vi "0506_Identificador_de_cor.vi"() -> (27 "error out":errorcluster)   [LabVIEW 2017]
uses:
  <vilib>/userdefined/High Color/IMAQdx.ctl
  <vilib>/vision/driver/IMAQdx.llb/IMAQdx Acquisition Mode.ctl
  <vilib>/vision/Classification.llb/IMAQ Classifier Read Options.ctl
  <vilib>/vision/driver/IMAQdx.llb/IMAQdx Buffer Number Mode.ctl
  <vilib>/vision/driver/NI_Vision_Acquisition_Software.lvlib
  <vilib>/vision/NI_Vision_Development_Module.lvlib
panel:
  out "Class":string
  out "dt":dbl
  out "Image Out 2":T1(plugin-control)
  in  "Câmera":T2="cam1"
  in  "Stop Button":bool
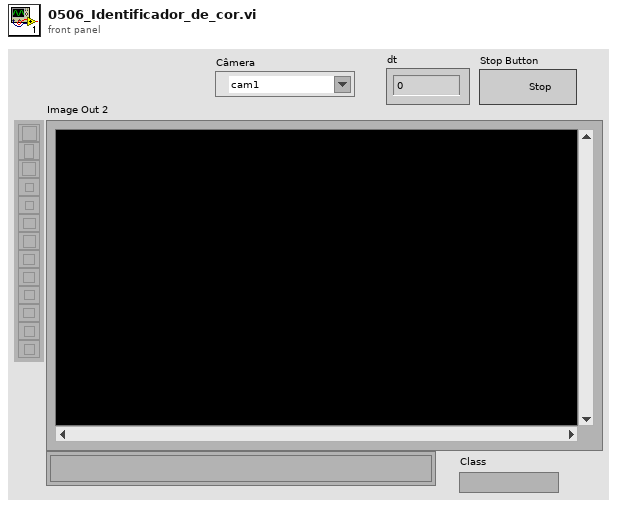
[diagram p1: front panel]
types:
  T1 = typedef "IMAQ Image.ctl" = refnum<image>
  T2 = typedef "IMAQdx.ctl" = refnum<k21>
  T3 = typedef "IMAQ Classifier Read Options.ctl" = i32
  T4 = typedef "Image Type" = u32
  T5 = typedef "NI_Vision_Acquisition_Software.lvlib/IMAQdx Acquisition Mode.ctl" = enum32{"One Shot", "Continuous"}
  T6 = typedef "IMAQ Classifier Session.ctl" = refnum<k1>
  T7 = typedef "NI_Vision_Acquisition_Software.lvlib/IMAQdx Buffer Number Mode.ctl" = enum32{"Next", "Last", "Buffer Number", "Every", "Last New"}
  T8 = cluster{"Global Rectangle":i32[], "Contours":cluster{"Contour Type":u32, "ROI Type":u32, "Points":i32[]}[]}
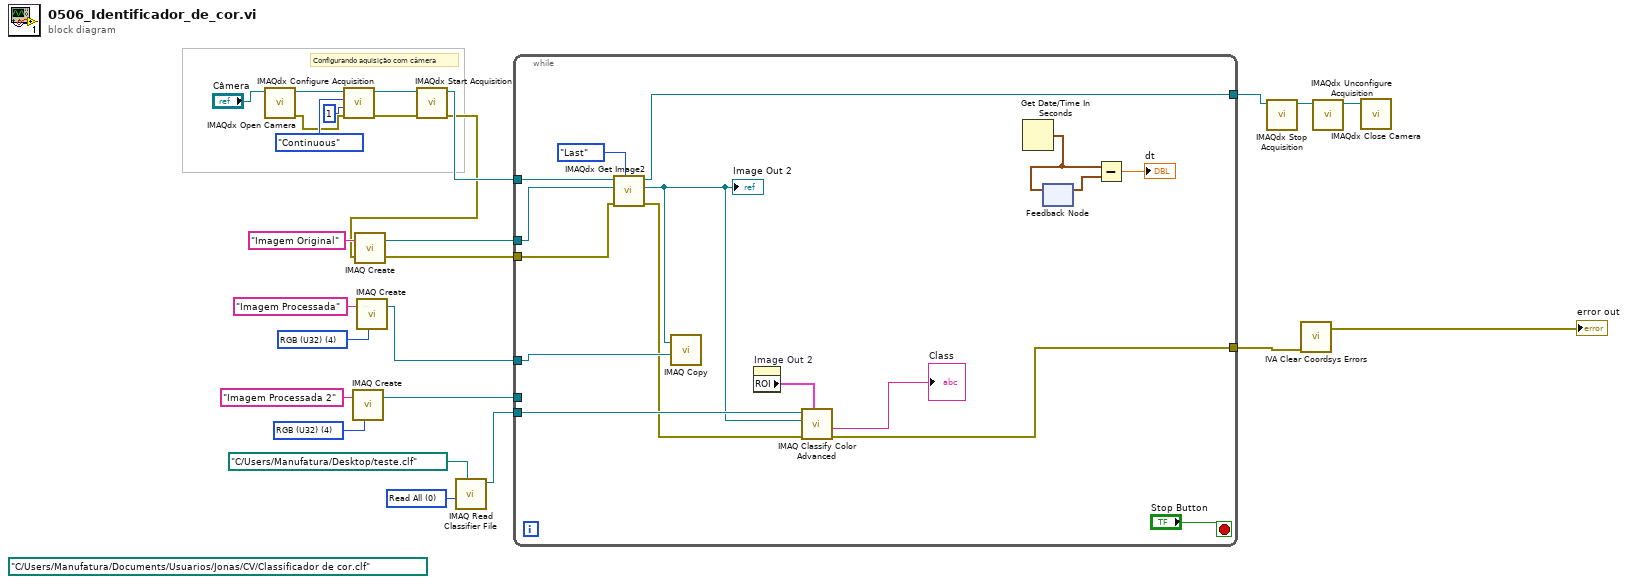
[diagram p0: block diagram]
diagram:
  (unwired) path "C:/Users/Manufatura/Documents/Usuarios/Jonas/CV/Classificador de cor.clf" ("File Path")
  w3 = T3 0 items=["Read All", "Add Samples, Do Not Change Options", "Read Options, Do Not Add Samples"] ("Read Options")
  w7 = T4 4 items=["Grayscale (U8)", "Grayscale (I16)", "Grayscale (SGL)", "Complex (CSG)", "RGB (U32)", "HSL (U32)", "RGB (U64)", "Grayscale (U16)"] ("Image Type")
  w20 = T4 4 items=["Grayscale (U8)", "Grayscale (I16)", "Grayscale (SGL)", "Complex (CSG)", "RGB (U32)", "HSL (U32)", "RGB (U64)", "Grayscale (U16)"] ("Image Type")
  # "Configurando aquisição com câmera"
  n1 = call <vilib>:"IMAQdx Open Camera.vi"("Session In"="Câmera") -> ("error out"=w16:errorcluster, "Session Out"=w26:T2)  [unwired: 9 in]
  n2 = call <vilib>:"IMAQdx Configure Acquisition.vi"("error in"=w16, "Number of Buffers"=u32 1, "Continuous?"=IMAQdx_Acquisition_Mode."Continuous", "Session In"=w26) -> ("error out"=w17:errorcluster, "Session Out"=w25:T2)  [unwired: 6 in]
  n3 = call "IMAQ Create"("Image Name"="Imagem Processada 2", "Image Type"=w7) -> ("New Image"=w5:T1)  [unwired: 3 in, 1 out]
  n4 = call "IMAQ Create"("Image Name"="Imagem Processada", "Image Type"=w20) -> ("New Image"=w8:T1)  [unwired: 3 in, 1 out]
  n5 = call <vilib>:"IMAQdx Start Acquisition.vi"("error in"=w17, "Session In"=w25) -> ("error out"=w15:errorcluster, "Session Out"=w18:T2)  [unwired: 8 in]
  n6 = call "IMAQ Create"("Image Name"="Imagem Original", "error in (no error)"=w15) -> ("New Image"=w19:T1, "error out"=w14:errorcluster)  [unwired: 3 in]
  n7 = call "IMAQ Read Classifier File"("File Path"=path "C:/Users/Manufatura/Desktop/teste.clf", "Read Options"=w3) -> ("Classifier Session"=w2:T6)  [unwired: 2 in, 7 out]
  n8 = while {
    tunnel: w19 -> [w41]
    tunnel: w18 -> [w40]
    tunnel: w14 -> [w39]
    tunnel: [w27] -> w13
    tunnel: [w37] -> w10
    tunnel: w8 -> [w36]
    tunnel: w5 -> [_]
    tunnel: w2 -> [w32]
    stop <- "Stop Button" stop-if-true
    n9 = call <vilib>:"IMAQdx Get Image2.vi"("Buffer Number Mode (Next)"=IMAQdx_Buffer_Number_Mode."Last", "error in"=w39, "Image In"=w41, "Session In"=w40) -> ("error out"=w30:errorcluster, "Image Out"=w31:T1, "Session Out"=w37:T2)  [unwired: 4 in, 1 out]
    "Image Out 2" <- w31
    n10 = call "IMAQ Copy"("Image Dst"=w36, "Image Src"=w31) -> ()  [unwired: 4 in, 2 out]
    n11 = property on="Image Out 2" class="ImageControl"() -> ("ROI"=w29:T8)  [unwired: 2 in, 2 out]
    n12 = call "IMAQ Classify Color Advanced"("ROI Descriptor"=w29, "error in (no error)"=w30, "Image"=w31, "Classifier Session"=w32) -> ("error out"=w27:errorcluster, "Class"=→"Class":string)  [unwired: 6 out]
    n13 = Get Date/Time In Seconds() -> (seconds since 1Jan1904=w34:timestamp)
    n14 = feedback #1() -> (w35:timestamp)  [unwired: 1 in]
    n15 = feedback-in #1(w34) -> ()
    n16 = Subtract(x=w34, y=w35) -> (x-y=→"dt":dbl)
  }
  n17 = call <vilib>:"IMAQdx Stop Acquisition.vi"("Session In"=w10) -> ("Session Out"=w12:T2)  [unwired: 9 in, 1 out]
  n18 = call <vilib>:"IVA Clear Coordsys Errors.vi"("error in (no error)"=w13) -> ("error out"=→"error out":errorcluster)  [unwired: 10 in]
  n19 = call <vilib>:"IMAQdx Unconfigure Acquisition.vi"("Session In"=w12) -> ("Session Out"=w11:T2)  [unwired: 9 in, 1 out]
  n20 = call <vilib>:"IMAQdx Close Camera.vi"("Session In"=w11) -> ()  [unwired: 10 in, 1 out]
